vi "HB_ThreadPool.MainLoopingTask_NInstrSim.vi"() -> ()   [LabVIEW 2009, in "HB_Device_Examples.lvlib"]
doc: "Simple application to test the HGF_ThreadPool with a simple class."
uses:
  HB_Device_Examples.lvlib
  NInstrSim/Factory/HB_DeviceFactory.lvclass
  lib.lib/HGF_LVC/HGF_BaseClasses/HGF_Factory/HGF_Factory.lvclass
  NInstrSim/Visitors/NInstrSim_ReadStatus/NInstrSim_ReadStatus.lvclass
  lib.lib/HGF_LVC/HGF_BaseClasses/HGF_Notifier/HGF_Notifier.lvclass
  NInstrSim/NInstrSim.lvclass
  lib.lib/HGF_LVC/HGF_BaseClasses/HGF_ThreadTask/HGF_ThreadTask.lvclass
  lib.lib/HGF_LVC/HGF_BaseClasses/HGF_Visitable/HGF_Visitable.lvclass
  lib.lib/HGF_LVC/HGF_BaseClasses/HGF_Queue/HGF_Queue.lvclass
  lib.lib/HGF_LVC/HGF_BaseClasses/HGF_Stop/HGF_Stop.lvclass
  lib.lib/HGF_LVC/HGF_BaseClasses/HGF_ThreadPool/HGF_ThreadPool.lvclass
  lib.lib/HGF_LVC/HGF_BaseClasses/HGF_Reference/HGF_Reference.lvclass
  lib.lib/HGF_LVC/HGF_BaseClasses/HGF_Event/HGF_Event.lvclass
  lib.lib/HGF_LVC/HGF_Auxiliary/HGF_Auxiliary.lvlib
  lib.lib/HGF_LVC/HGF_DeviceBaseClasses/HGF_VISADevice/HGF_VISADevice.lvclass
  lib.lib/HGF_LVC/HGF_DeviceBaseClasses/HGF_DeviceBase/HGF_DeviceBase.lvclass
  lib.lib/HGF_LVC/HGF_BaseClasses/HGF_Timing/HGF_Timing.lvclass
  NInstrSim/Visitors/NInstrSim_ConfigureWaveformType/NInstrSim_ConfigureWaveformType.lvclass
panel:
  out "found?":bool
  out "error?":bool
  out "objectErrors":errorcluster[](array[cluster])
  out "dcMeasurement":dbl format="%_6g"
  out "Waveform Graph":waveform(dbl)(graph)
  in  "function (0:Sine)":u16(ring) items=["Sine", "Square", "Sine+Noise", "Random", "Chirp"]
  in  "VISA Resource Name":refnum<visa-resource-name>
  in  "Serial Configuration":T1={"Baud Rate"=9600, "Flow Control"=0, "Parity"=0, "Data Bits"=8, "Stop Bits"=10} {"Stop Bits" items=["1.0"=10, "1.5"=15, "2.0"=20]; "Data Bits" items=["7"=7, "8"=8]; "Parity" items=["None", "Odd", "Even", "Mark", "Space"]; "Flow Control" items=["None"=0, "XON/XOFF"=1, "RTS/CTS"=2, "DTR/DSR"=4]; "Baud Rate" items=["300"=300, "600"=600, "1200"=1200, "2400"=2400, "4800"=4800, "9600"=9600, "19200"=19200]}
  in  "timeout in ms (-1)":i32=3000
  out "nofTasksInQueueOut":i32
  out "nofTasksWaiting":i32
  out "autoIncrementLimit":i32=-1
  out "nofThreads":i32
  out "Default Destination timed out?":bool
  out "got object?":bool
  out "commandError":errorcluster
  in  "stop":bool
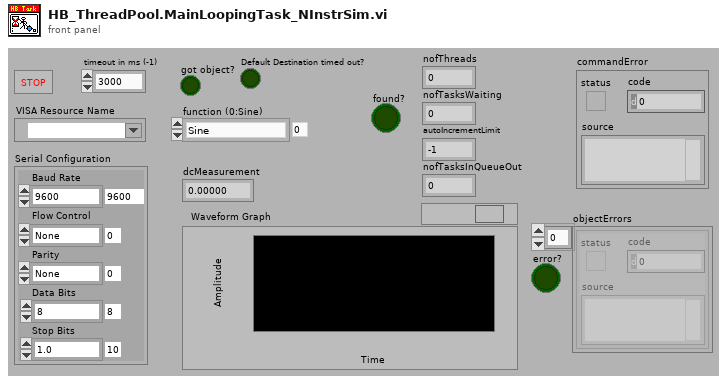
[diagram p1: front panel]
types:
  T1 = cluster{"Baud Rate":u32, "Flow Control":u16, "Parity":u16, "Data Bits":u16, "Stop Bits":u16}
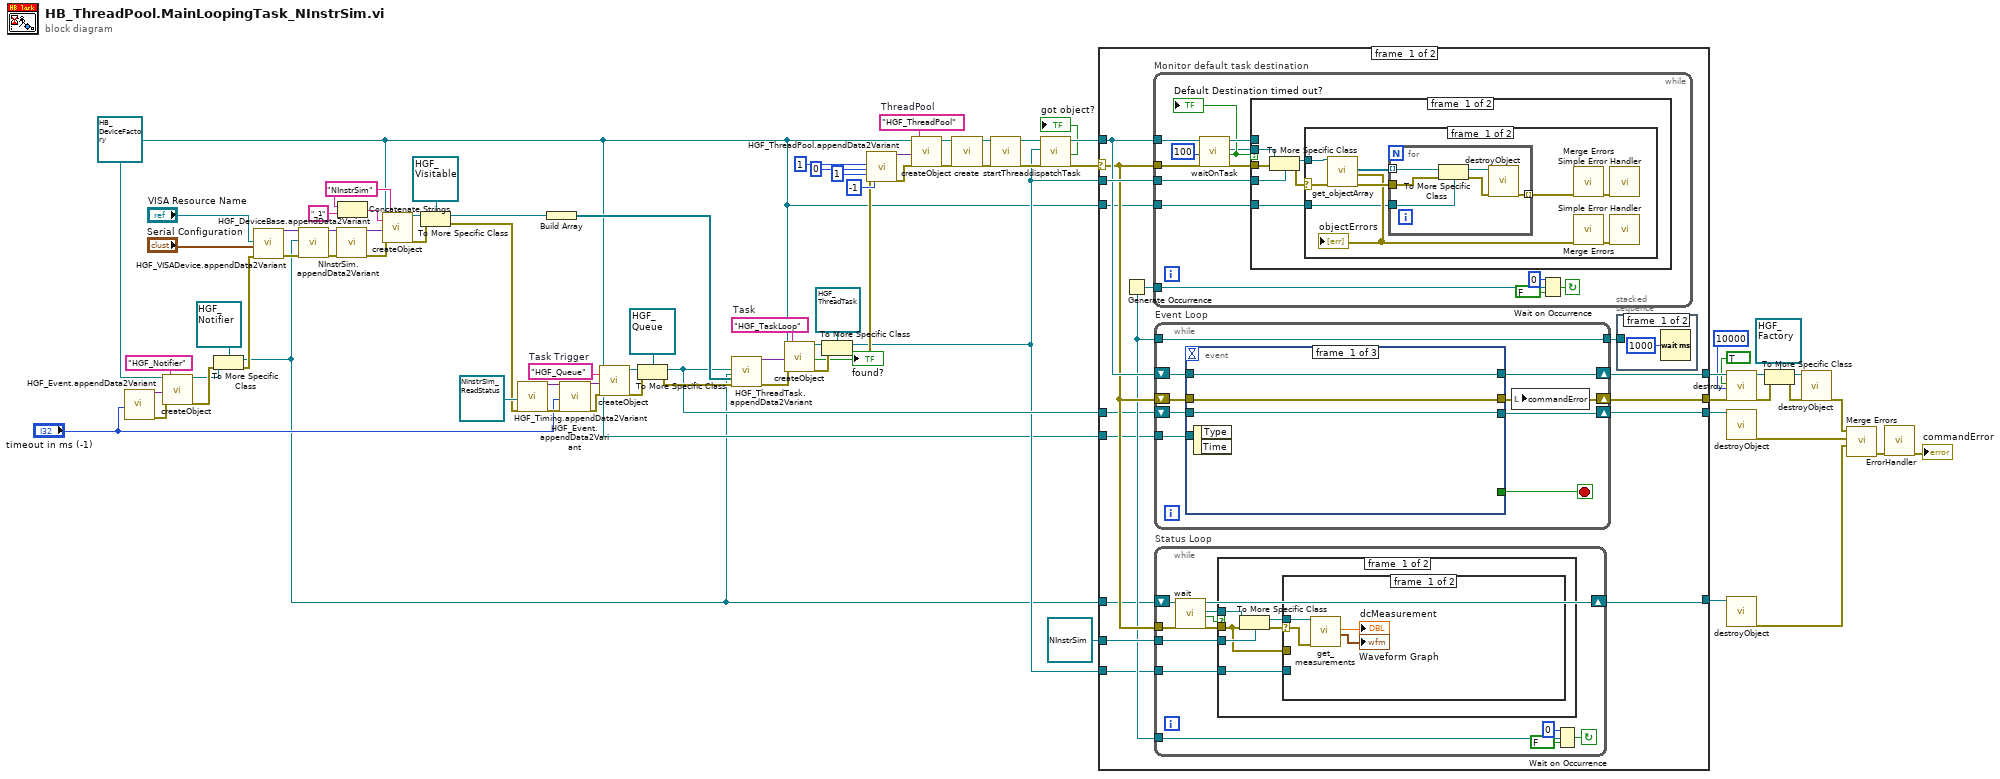
[diagram p0: block diagram]
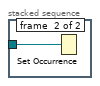
[diagram p2: hidden frame]
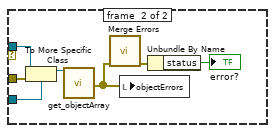
[diagram p3: hidden frame]
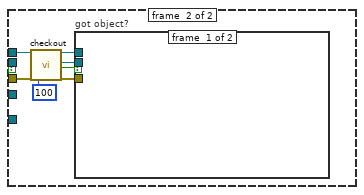
[diagram p6: hidden frame]
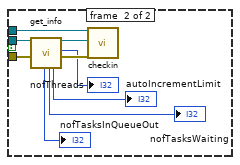
[diagram p7: hidden frame]
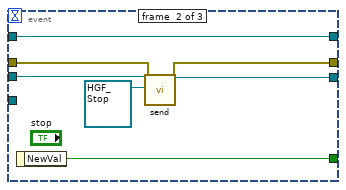
[diagram p8: hidden frame]
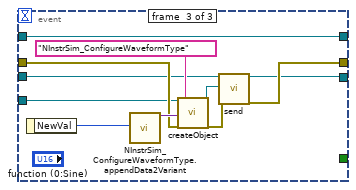
[diagram p9: hidden frame]
diagram:
  w46 = "NInstrSim" ("className")
  w61 = "HGF_Queue"  # Task Trigger
  w60 = "HGF_TaskLoop"  # Task
  w52 = "HGF_ThreadPool"  # ThreadPool
  w5 = refnum<class "HB_DeviceFactory.lvclass"> refnum ("HB_Factory.lvclass")
  n1 = call "HGF_Event.appendData2Variant.vi"("timeout in ms (-1)"="timeout in ms (-1)") -> ("dup initData"=w27:variant, "error out"=w28:errorcluster)  [unwired: 2 in, 15 out]
  n2 = call "createObject.vi"("HGF_Factory"=w5, "initializationData"=w27, "error in (no error)"=w28, "className"="HGF_Notifier") -> ("HGF_Object"=w24:refnum<class "HGF_Factory.lvclass">, "error out"=w25:errorcluster)  [unwired: 2 in, 12 out]
  n3 = To More Specific Class(target class=refnum<class "HGF_Notifier.lvclass"> refnum ("HGF_BaseClasses.lvlib:HGF_Notifier.lvclass"), reference=w24, error in=w25) -> (specific class reference=w3:refnum<class "HGF_Notifier.lvclass">, error out=w23:errorcluster)
  n4 = call "HGF_VISADevice.appendData2Variant.vi"("VISA Resource Name"="VISA Resource Name", "Serial Configuration"="Serial Configuration", "error in (no error)"=w23) -> ("dup initData"=w32:variant, "error out"=w30:errorcluster)  [unwired: 1 in, 14 out]
  n5 = call "NInstrSim.appendData2Variant.vi"("initData"=w32, "statusEvent"=w3, "error in (no error)"=w30) -> ("dup initData"=w31:variant, "error out"=w29:errorcluster)  [unwired: 15 out]
  n6 = call "HGF_DeviceBase.appendData2Variant.vi"("initData"=w31, "error in (no error)"=w29) -> ("dup initData"=w47:variant, "error out"=w19:errorcluster)  [unwired: 16 out]
  n7 = Concatenate Strings(w46, "_1" ("string")) -> (w44:string)
  n8 = call "createObject.vi"("HGF_Factory"=w5, "objectName"=w44, "initializationData"=w47, "error in (no error)"=w19, "className"=w46) -> ("HGF_Object"=w50:refnum<class "HGF_Factory.lvclass">, "error out"=w51:errorcluster)  [unwired: 1 in, 12 out]
  n9 = To More Specific Class(target class=refnum<class "HGF_Visitable.lvclass"> refnum ("HGF_BaseClasses.lvlib:HGF_Visitable.lvclass"), reference=w50, error in=w51) -> (specific class reference=w65:refnum<class "HGF_Visitable.lvclass">, error out=w16:errorcluster)
  n10 = call "HGF_Timing.appendData2Variant.vi"("defaultObject"=refnum<class "NInstrSim_ReadStatus.lvclass"> refnum ("HB_HGF_Test.lvlib:NInstrSim_ReadStatus.lvclass"), "error in (no error)"=w16) -> ("dup initData"=w36:variant, "error out"=w35:errorcluster)  [unwired: 1 in, 15 out]
  n11 = Build Array(w65) -> (w42:refnum<class "HGF_Visitable.lvclass">[])
  n12 = call "HGF_Event.appendData2Variant.vi"("initData"=w36, "timeout in ms (-1)"="timeout in ms (-1)", "error in (no error)"=w35) -> ("dup initData"=w67:variant, "error out"=w66:errorcluster)  [unwired: 1 in, 14 out]
  n13 = call "createObject.vi"("HGF_Factory"=w5, "initializationData"=w67, "error in (no error)"=w66, "className"=w61) -> ("HGF_Object"=w58:refnum<class "HGF_Factory.lvclass">, "error out"=w68:errorcluster)  [unwired: 2 in, 12 out]
  n14 = To More Specific Class(target class=refnum<class "HGF_Queue.lvclass"> refnum ("HGF_BaseClasses.lvlib:HGF_Queue.lvclass"), reference=w58, error in=w68) -> (specific class reference=w33:refnum<class "HGF_Queue.lvclass">, error out=w43:errorcluster)
  n15 = call "HGF_ThreadTask.appendData2Variant.vi"("taskTrigger"=w33, "taskDestination"=w3, "objectArray"=w42, "error in (no error)"=w43) -> ("dup initData"=w2:variant, "error out"=w1:errorcluster)  [unwired: 2 in, 12 out]
  n16 = call "createObject.vi"("HGF_Factory"=w5, "initializationData"=w2, "error in (no error)"=w1, "className"=w60) -> ("HGF_Object"=w57:refnum<class "HGF_Factory.lvclass">, "found?"=→"found?":bool, "error out"=w64:errorcluster)  [unwired: 2 in, 11 out]
  n17 = To More Specific Class(target class=refnum<class "HGF_ThreadTask.lvclass"> refnum ("HGF_BaseClasses.lvlib:HGF_ThreadTask.lvclass"), reference=w57, error in=w64) -> (specific class reference=w12:refnum<class "HGF_ThreadTask.lvclass">, error out=w17:errorcluster)
  n18 = call "HGF_ThreadPool.appendData2Variant.vi"("initialNofThreads (0)"=1 ("initialNofThreads"), "incThreads(1)"=0 ("incThreads"), "maxNofThreads (-1:unlimited)"=1 ("maxNofThreads"), "error in (no error)"=w17, "autoIncrementLimit (-1)"=-1) -> ("dup initData"=w79:variant, "error out"=w18:errorcluster)  [unwired: 2 in, 11 out]
  n19 = call "createObject.vi"("HGF_Factory"=w5, "initializationData"=w79, "error in (no error)"=w18, "className"=w52) -> ("HGF_Object"=w59:refnum<class "HGF_Factory.lvclass">, "error out"=w78:errorcluster)  [unwired: 2 in, 12 out]
  n20 = call "create.vi"("Object"=w59, "error in (no error)"=w78) -> ("HGF_Reference"=w80:refnum<class "HGF_Reference.lvclass">, "error out"=w74:errorcluster)  [unwired: 1 in, 15 out]
  n21 = call "startThread.vi"("HGF_ThreadPool_Reference"=w80, "error in (no error)"=w74) -> ("dup HGF_ThreadPool_Reference"=w41:refnum<class "HGF_Reference.lvclass">, "error out"=w39:errorcluster)  [unwired: 1 in, 15 out]
  n22 = call "dispatchTask.vi"("HGF_ThreadPool_Reference"=w41, "HGF_ThreadTask"=w12, "error in (no error)"=w39) -> ("dup HGF_ThreadPool_Reference"=w40:refnum<class "HGF_Reference.lvclass">, "got object?"=→"got object?":bool, "error out"=w38:errorcluster)  [unwired: 1 in, 13 out]
  n23 = case shown="No Error" w38 {
    selector: w38 -> [w90 w209]
    tunnel: w40 -> [w92 w210]
    tunnel: [w95 w210] -> w63
    tunnel: w12 -> [w93 _]
    tunnel: [w94 w209] -> w62
    tunnel: w33 -> [w84 w207]
    tunnel: w3 -> [w86 w208]
    tunnel: refnum<class "NInstrSim.lvclass"> refnum ("HB_HGF_Test.lvlib:NInstrSim.lvclass") -> [w89 _]
    tunnel: w5 -> [w87 _]
    tunnel: [w83 w208] -> w14
    tunnel: w12 -> [w85 _]
    tunnel: [w82 w207] -> w10
    tunnel: w5 -> [w81 _]
    frame #0 {
      n24 = Generate Occurrence() -> (w88:refnum<k4>)
      n25 = while "Monitor default task destination" {
        tunnel: w93 -> [w135]
        tunnel: w92 -> [w134]
        tunnel: w90 -> [w133]
        tunnel: w88 -> [w128]
        tunnel: w81 -> [w127]
        stop <- w129 continue-if-true
        n26 = call "waitOnTask.vi"("HGF_ThreadPool_Reference"=w134, "timeout in ms (-1)"=100, "error in (no error)"=w133) -> ("dup HGF_ThreadPool_Reference"=w139:refnum<class "HGF_Reference.lvclass">, "HGF_Task"=w137:refnum<class "HGF_ThreadTask.lvclass">, "timed out?"=w138:bool, "error out"=w132:errorcluster)  [unwired: 13 out]
        "Default Destination timed out?" <- w138
        n27 = case "timed out?" shown="False" w138 {
          tunnel: w137 -> [w145 _]
          tunnel: w132 -> [w144 w161]
          tunnel: w139 -> [_ w162]
          tunnel: w135 -> [w141 _]
          tunnel: w127 -> [w140 _]
          frame #0 {
            n28 = To More Specific Class(target class=w141, reference=w145, error in=w144) -> (specific class reference=w143:refnum<class "HGF_ThreadTask.lvclass">, error out=w142:errorcluster)
            n29 = case shown="No Error" w142 {
              selector: w142 -> [w153 _]
              tunnel: w143 -> [w154 _]
              tunnel: w140 -> [w146 _]
              frame #0 {
                n30 = call "get_objectArray.vi"("HGF_ThreadTask"=w154, "error in (no error)"=w153) -> ("objectArray"=w149:refnum<class>[], "errorArray"=w147:errorcluster[], "error out"=w151:errorcluster)  [unwired: 15 out]
                "objectErrors" <- w147
                n31 = for {
                  tunnel: w151 -> [w157]
                  tunnel: [w160] -> w152 mode=indexing
                  tunnel: w149 -> [w159] mode=indexing
                  tunnel: w146 -> [w155]
                  n32 = To More Specific Class(target class=w155, reference=w159, error in=w157) -> (specific class reference=w158:refnum<class "HB_DeviceFactory.lvclass">, error out=w156:errorcluster)
                  n33 = call "destroyObject.vi"("HGF_Factory"=w158, "error in (no error)"=w156) -> ("error out"=w160:errorcluster)  [unwired: 17 out]
                }
                n34 = call <vilib>:"Merge Errors.vi"("error array in"=w152) -> ("error out"=w150:errorcluster)  [unwired: 3 in, 3 out]
                n35 = call <vilib>:"Merge Errors.vi"("error array in"=w147) -> ("error out"=w148:errorcluster)  [unwired: 3 in, 3 out]
                n36 = call <vilib>:"Simple Error Handler.vi"("error in (no error)"=w150) -> ()  [unwired: 1 in, 8 out]
                n37 = call <vilib>:"Simple Error Handler.vi"("error in (no error)"=w148) -> ()  [unwired: 1 in, 8 out]
              }
              frame #1 {
              }
            }
          }
          frame #1 {
            n38 = call "checkout.vi"("HGF_ThreadPool_Reference"=w162, "timeout in ms (-1)"=100, "error in (no error)"=w161) -> ("dup HGF_ThreadPool_Reference"=w163:refnum<class "HGF_Reference.lvclass">, "HGF_ThreadPool"=w164:refnum<class "HGF_ThreadPool.lvclass">, "got object?"=w167:bool, "error out"=w165:errorcluster)  [unwired: 13 out]
            n39 = case "got object?" shown="True" w167 {
              tunnel: w163 -> [_ w176]
              tunnel: w164 -> [_ w175]
              tunnel: w165 -> [_ w174]
              frame #0 {
              }
              frame #1 {
                n40 = call "get_info.vi"("HGF_ThreadPool"=w175, "error in (no error)"=w174) -> ("nofTasksInQueueOut"=→"nofTasksInQueueOut":i32, "nofTasksWaiting"=→"nofTasksWaiting":i32, "autoIncrementLimit"=→"autoIncrementLimit":i32, "dup HGF_ThreadPool"=w172:refnum<class "HGF_ThreadPool.lvclass">, "nofThreads"=→"nofThreads":i32, "error out"=w173:errorcluster)  [unwired: 12 out]
                n41 = call "checkin.vi"("HGF_Reference"=w176, "Object"=w172, "error in (no error)"=w173) -> ()  [unwired: 1 in, 16 out]
              }
            }
          }
        }
        n42 = Wait on Occurrence(1:FALSE ("ignore previous (T)"), 2:w128, 3:0 ("ms timeout (-1)")) -> (0:w129:bool)
      }
      n43 = while "Event Loop" {
        shift-right: [w184] -> w95
        shift-left: w92 -> [w183]
        shift-right: [w180] -> w94
        shift-left: w90 -> [w185]
        tunnel: w88 -> [w179]
        tunnel: [w179] -> w91
        tunnel: w87 -> [w181]
        shift-right: [w177] -> w82
        shift-left: w84 -> [w182]
        stop <- w178 stop-if-true
        n44 = event shown="[2] \"function (0:Sine)\": Value Change" {
          selector: _ -> [_ _ _]
          dyn-events: _ -> [_ _ _]
          timeout: _ -> [_ _ _]
          tunnel: [_ w195 _] -> w178
          tunnel: [w187 w190 w198] -> w180
          tunnel: w185 -> [w187 w191 w203]
          tunnel: [w188 w194 w206] -> w184
          tunnel: w183 -> [w188 w194 w206]
          tunnel: w182 -> [w186 w193 w201]
          tunnel: w181 -> [_ _ w197]
          tunnel: [w186 w189 w196] -> w177
          event #0 {
            n45 = event-data() -> ()  [unwired: 3 out]
          }
          event #1 {
            n46 = event-data() -> ("NewVal"=w195:bool)  [unwired: 1 out]
            n47 = call-dynamic "send.vi"("HGF_Queue"=w193, "Object"=refnum<class "HGF_Stop.lvclass"> refnum ("HGF_BaseClasses.lvlib:HGF_Stop.lvclass"), "error in (no error)"=w191) -> ("HGF_Queue"=w189:refnum<class "HGF_Queue.lvclass">, "error out"=w190:errorcluster)  [unwired: 2 in, 13 out]
          }
          event #2 {
            n48 = event-data() -> ("NewVal"=w202:u16)  [unwired: 1 out]
            n49 = call "NInstrSim_ConfigureWaveformType.appendData2Variant.vi"("function (0:Sine)"=w202) -> ("dup initData"=w205:variant)  [unwired: 2 in, 16 out]
            n50 = call "createObject.vi"("HGF_Factory"=w197, "initializationData"=w205, "error in (no error)"=w203, "className"="NInstrSim_ConfigureWaveformType") -> ("HGF_Object"=w200:refnum<class "HGF_Factory.lvclass">, "error out"=w199:errorcluster)  [unwired: 2 in, 12 out]
            n51 = call-dynamic "send.vi"("HGF_Queue"=w201, "Object"=w200, "error in (no error)"=w199) -> ("HGF_Queue"=w196:refnum<class "HGF_Queue.lvclass">, "error out"=w198:errorcluster)  [unwired: 2 in, 13 out]
          }
        }
        n52 = local write "commandError"(w180) -> ()
      }
      n53 = while "Status Loop" {
        tunnel: w90 -> [w108]
        tunnel: w89 -> [w105]
        tunnel: w88 -> [w100]
        tunnel: w85 -> [w99]
        shift-right: [w98] -> w83
        shift-left: w86 -> [w109]
        stop <- w101 continue-if-true
        n54 = call-dynamic "wait.vi"("HGF_Notifier"=w109, "error in (no error)"=w108) -> ("dup HGF_Notifier"=w98:refnum<class "HGF_Notifier.lvclass">, "Object"=w106:refnum<class>, "timed out"=w104:bool, "error out"=w107:errorcluster)  [unwired: 2 in, 12 out]
        n55 = case shown="True" w104 {
          tunnel: w107 -> [w111 _]
          tunnel: w106 -> [w115 _]
          tunnel: w105 -> [w114 _]
          tunnel: w99 -> [w110 _]
          frame #0 {
            n56 = To More Specific Class(target class=w114, reference=w115, error in=w111) -> (specific class reference=w112:refnum<class "NInstrSim.lvclass">, error out=w113:errorcluster)
            n57 = case shown="No Error" w113 {
              selector: w113 -> [w119 _]
              tunnel: w112 -> [w118 w126]
              tunnel: w111 -> [_ w125]
              tunnel: w110 -> [_ w124]
              frame #0 {
                n58 = call "get_measurements.vi"("NInstrSim"=w118, "error in (no error)"=w119) -> ("dcMeasurement"=→"dcMeasurement":dbl, "waveform"=→"Waveform Graph":waveform(dbl))  [unwired: 16 out]
              }
              frame #1 {
                n59 = To More Specific Class(target class=w124, reference=w126, error in=w125) -> (specific class reference=w123:refnum<class "HGF_ThreadTask.lvclass">)  [unwired: 1 out]
                n60 = call "get_objectArray.vi"("HGF_ThreadTask"=w123) -> ("errorArray"=w122:errorcluster[])  [unwired: 1 in, 17 out]
                n61 = call <vilib>:"Merge Errors.vi"("error array in"=w122) -> ("error out"=w121:errorcluster)  [unwired: 3 in, 3 out]
                n62 = local write "objectErrors"(w122) -> ()
                n63 = Unbundle By Name(w121) -> ("status"=→"error?":bool)
              }
            }
          }
          frame #1 {
          }
        }
        n64 = Wait on Occurrence(1:FALSE ("ignore previous (T)"), 2:w100, 3:0 ("ms timeout (-1)")) -> (0:w101:bool)
      }
      n65 = stacked-sequence {
        tunnel: w91 -> [_ w97]
        frame #0 {
          n66 = Wait (ms)(milliseconds to wait=u32 1000) -> ()  [unwired: 1 out]
        }
        frame #1 {
          n67 = Set Occurrence(w97) -> ()
        }
      }
    }
    frame #1 {
    }
  }
  n68 = call "destroy.vi"("HGF_Reference"=w63, "wait for activity? (F)"=TRUE, "timeout /ms (-1)"=10000, "error in (no error)"=w62) -> ("Object"=w73:refnum<class>, "error out"=w71:errorcluster)  [unwired: 14 out]
  n69 = call "destroyObject.vi"("HGF_Factory"=w10) -> ("error out"=w7:errorcluster)  [unwired: 1 in, 17 out]
  n70 = call "destroyObject.vi"("HGF_Factory"=w14) -> ("error out"=w6:errorcluster)  [unwired: 1 in, 17 out]
  n71 = To More Specific Class(target class=refnum<class "HGF_Factory.lvclass"> refnum ("HGF_BaseClasses.lvlib:HGF_Factory.lvclass"), reference=w73, error in=w71) -> (specific class reference=w72:refnum<class "HGF_Factory.lvclass">, error out=w70:errorcluster)
  n72 = call "destroyObject.vi"("HGF_Factory"=w72, "error in (no error)"=w70) -> ("error out"=w9:errorcluster)  [unwired: 17 out]
  n73 = call <vilib>:"Merge Errors.vi"("error in 3 (no error)"=w6, "error in 2 (no error)"=w7, "error in 1 (no error)"=w9) -> ("error out"=w8:errorcluster)  [unwired: 1 in, 3 out]
  n74 = call "ErrorHandler.vi"("error in (no error)"=w8) -> ("error out"=→"commandError":errorcluster)  [unwired: 6 in, 12 out]
